vi "Fuse 10.vi"() -> ()   [LabVIEW 2014]
uses:
  <instrlib>/niDMM/nidmm.llb/niDMM Configure Measurement Absolute.vi
  <instrlib>/niDMM/nidmm.llb/niDMM Function.ctl
panel:
  out "Time to Switch 2":dbl format="%#_12g"
  out "relative seconds 2":dbl format="%_19f"
  out "relative seconds":dbl format="%_19f"
  out "End time 2":timestamp format="%<%.6X>T"
  out "Output Current":dbl format="%.4f"
  out "Measurement":dbl format="%.5f"
  out "End time":timestamp format="%<%.6X>T"
  out "val change ind":bool
  out "error out":errorcluster
  out "Start Time":timestamp format="%<%.6X>T"
  in  "Output On/Off":bool
  out "Time to Switch":dbl format="%#_12g"
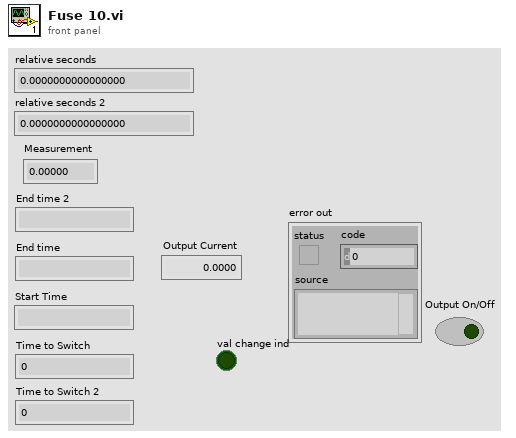
[diagram p1: front panel]
types:
  T1 = typedef "niDMM Function.ctl" = enum16{"DC Volts", "AC Volts", "DC Current", "AC Current", "2-wire Resistance", "4-wire Resistance", "Diode", "Frequency", "Period", "AC Volts DC Coupled", "Capacitance", "Inductance", "Temperature"}
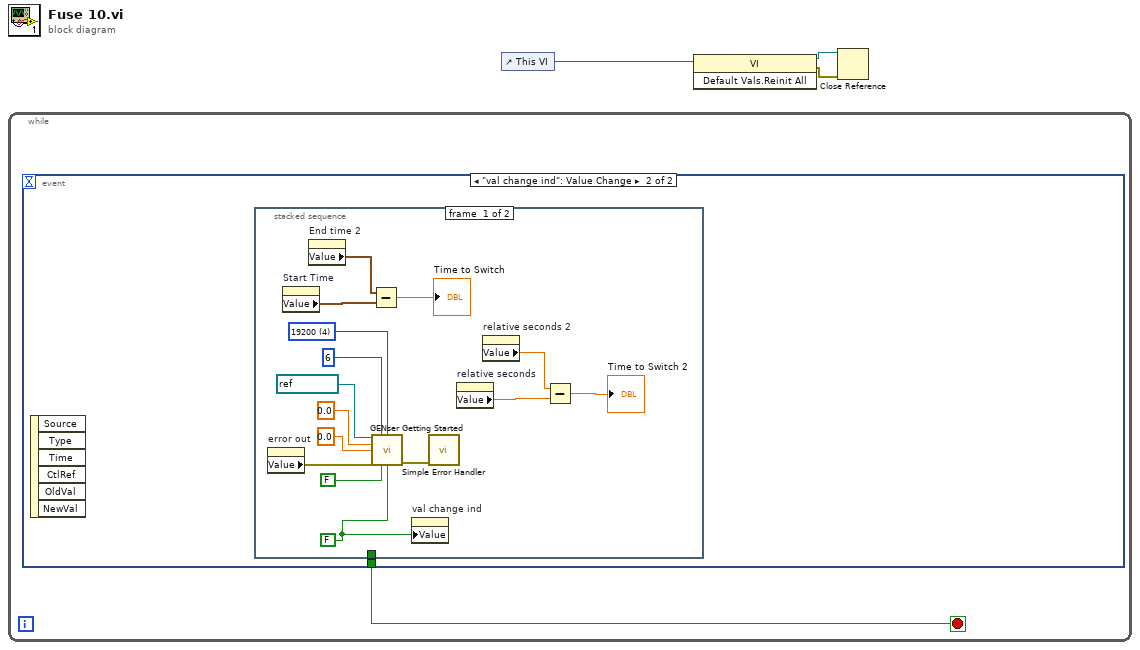
[diagram p0: block diagram]
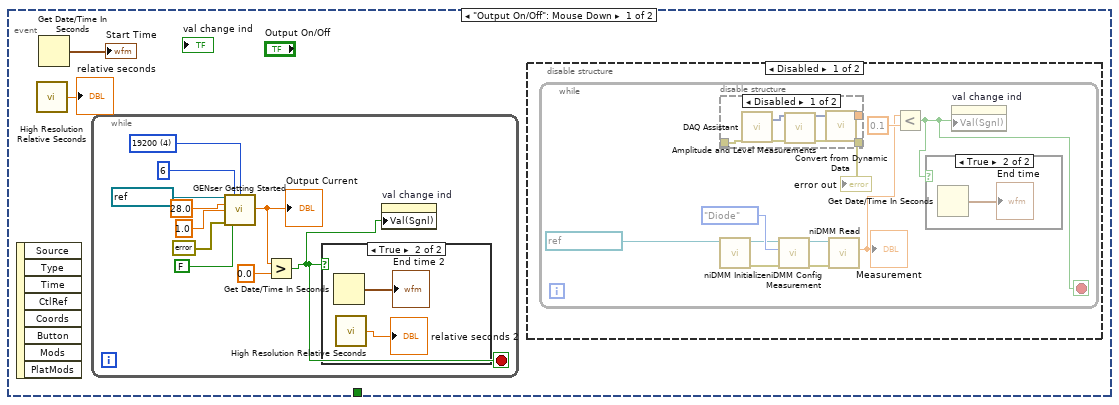
[diagram p2: hidden frame]
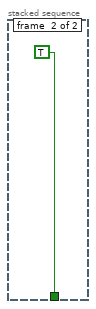
[diagram p7: hidden frame]
diagram:
  n1 = while {
    stop <- w4 stop-if-true
    n2 = event shown="[1] \"val change ind\": Value Change" {
      selector: _ -> [_ _]
      dyn-events: _ -> [_ _]
      timeout: _ -> [_ _]
      tunnel: [_ w36] -> w4
      event "Output On/Off": Mouse Down {
        n3 = event-data() -> ()  [unwired: 1 in, 8 out]
        n4 = call <vilib>:"High Resolution Relative Seconds.vi"() -> ("relative seconds"=→"relative seconds":dbl)
        n5 = Get Date/Time In Seconds() -> (seconds since 1Jan1904=→"Start Time":timestamp)
        n6 = while {
          stop <- w7 stop-if-true
          w15 = u16 4 items=["1200", "2400", "4800", "9600", "19200"] ("BAUD")
          n7 = call "GENser Getting Started.vi"("VISA"=refnum<visa-resource-name> "COM6", "GEN Addr"=i16 6, "BAUD"=w15, "Voltage Limit"=28.0, "Current Limit"=1.0, "error"=errorcluster {"status"=FALSE, "code"=0, "source"=""}, "Reset (T)"=FALSE) -> ("Output Current"=w10:dbl)  [unwired: 5 in, 3 out]
          "Output Current" <- w10
          n8 = Greater?(x=w10, y=0.0) -> (0:w7:bool)
          n9 = case shown="True" w7 {
            frame False {
            }
            frame True {
              n10 = Get Date/Time In Seconds() -> (seconds since 1Jan1904=→"End time 2":timestamp)
              n11 = call <vilib>:"High Resolution Relative Seconds.vi"() -> ("relative seconds"=→"relative seconds 2":dbl)
            }
          }
          n12 = property on="val change ind" class="Bool (strict)"("Val(Sgnl)"=w7) -> ()  [unwired: 2 in, 2 out]
        }
        n13 = disable-structure shown="Disabled" {
          frame Disabled {
            n14 = while {
              stop <- w26 stop-if-true
              n15 = call <instrlib>:"niDMM Initialize.vi"("Instrument Descriptor"=refnum<k15> "PXI1Slot9") -> ("error out"=w20:errorcluster, "instrument handle out"=w21:refnum<k15>)  [unwired: 9 in]
              n16 = disable-structure shown="Disabled" {
                disable-tunnel: [w34 _] -> w28
                disable-tunnel: [w32 _] -> _
                disable-tunnel: _ -> [w29 _]
                frame Disabled {
                  n17 = call "DAQ Assistant"("error in"=w29) -> ("data"=w33:dynamicdata, "error out"=w31:errorcluster)  [unwired: 16 in, 1 out]
                  n18 = call "Amplitude and Level Measurements"("Signals"=w33, "error in (no error)"=w31) -> ("Mean (DC)"=w30:dynamicdata, "error out"=w34:errorcluster)  [unwired: 12 in]
                  n19 = call "Convert from Dynamic Data"("Dynamic Data Type"=w30) -> ("Scalar"=w32:dbl)  [unwired: 3 in]
                }
                frame Enabled {
                }
              }
              "error out" <- w28
              n20 = call-poly <instrlib>:"niDMM Config Measurement.vi"("error in (no error)"=w20, "Function"=niDMM_Function."Diode", "instrument handle"=w21) -> ("error out"=w22:errorcluster, "instrument handle out"=w23:refnum<k15>)  [unwired: 7 in]
              n21 = call <instrlib>:"niDMM Read.vi"("error in (no error)"=w22, "instrument handle"=w23) -> ("Measurement"=w19:dbl)  [unwired: 7 in, 2 out]
              "Measurement" <- w19
              n22 = Less?(x=w19, y=0.1) -> (x < y?=w26:bool)
              n23 = case shown="True" w26 {
                frame False {
                }
                frame True {
                  n24 = Get Date/Time In Seconds() -> (seconds since 1Jan1904=→"End time":timestamp)
                }
              }
              n25 = property on="val change ind" class="Bool (strict)"("Val(Sgnl)"=w26) -> ()  [unwired: 2 in, 2 out]
            }
          }
          frame Enabled {
          }
        }
      }
      event "val change ind": Value Change {
        n26 = event-data() -> ()  [unwired: 1 in, 6 out]
        n27 = stacked-sequence {
          tunnel: [_ TRUE] -> w36
          frame #0 {
            w41 = FALSE
            w45 = u16 4 items=["1200", "2400", "4800", "9600", "19200"] ("BAUD")
            n28 = property on="error out" class="Clust (strict)"() -> ("Value"=w43:errorcluster)  [unwired: 2 in, 2 out]
            n29 = property on="Start Time" class="AbsTime (strict)"() -> ("Value"=w50:timestamp)  [unwired: 2 in, 2 out]
            n30 = property on="End time 2" class="AbsTime (strict)"() -> ("Value"=w40:timestamp)  [unwired: 2 in, 2 out]
            n31 = Subtract(x=w40, y=w50) -> (x-y=→"Time to Switch":dbl)
            n32 = call "GENser Getting Started.vi"("VISA"=refnum<visa-resource-name> "COM6", "GEN Addr"=i16 6, "BAUD"=w45, "Voltage Limit"=0.0, "Current Limit"=0.0, "error"=w43, "Reset (T)"=FALSE, "Output On (T)"=w41) -> ("error out"=w42:errorcluster)  [unwired: 4 in, 3 out]
            n33 = property on="val change ind" class="Bool (strict)"("Value"=w41) -> ()  [unwired: 2 in, 2 out]
            n34 = call <vilib>:"Simple Error Handler.vi"("error in (no error)"=w42) -> ()  [unwired: 4 in, 5 out]
            n35 = property on="relative seconds" class="DigNum (strict)"() -> ("Value"=w38:dbl)  [unwired: 2 in, 2 out]
            n36 = property on="relative seconds 2" class="DigNum (strict)"() -> ("Value"=w39:dbl)  [unwired: 2 in, 2 out]
            n37 = Subtract(x=w39, y=w38) -> (x-y=→"Time to Switch 2":dbl)
          }
          frame #1 {
          }
        }
      }
    }
  }
  n38 = control-ref of="This VI"() -> (w3:refnum<vi>)
  n39 = invoke class="VI" method="Default Vals.Reinit All"(reference=w3) -> (reference out=w1:refnum<vi>, error out=w2:errorcluster)  [unwired: 2 in, 1 out]
  n40 = Close Reference(reference=w1, error in (no error)=w2) -> ()  [unwired: 1 out]
